vi "SetVIActivationEvent.vi"(8 "error in (no error)":errorcluster, 10 "VIActivation":refnum<user-event>, 11 "VI Activation in":refnum<class "VIActivation.lvclass">) -> (0 "error out":errorcluster, 3 "VI Activation out":refnum<class "VIActivation.lvclass">)   [LabVIEW 2021, in "VIActivation.lvlib" / "VIActivation.lvclass"]
uses:
  VIActivation.lvclass
  VIActivation.lvclass/VIActivation.ctl
  VIActivationEvents.ctl
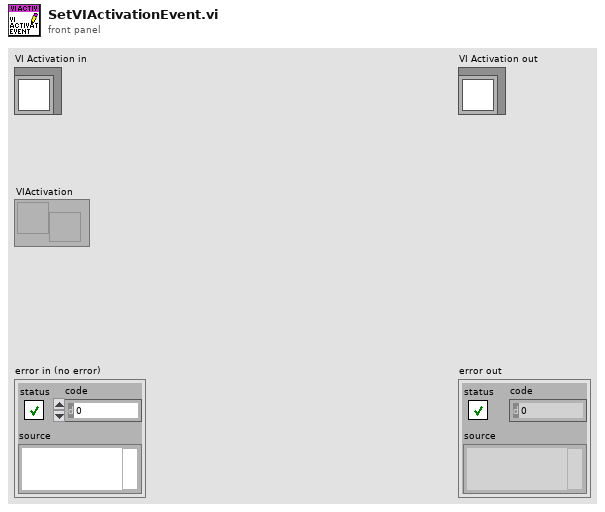
[diagram p1: front panel]
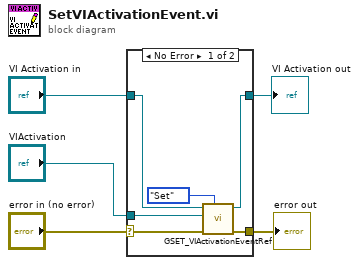
[diagram p0: block diagram]
diagram:
  n1 = case shown="No Error" "error in (no error)" {
    selector: "error in (no error)" -> [w11 w13]
    tunnel: [w10 w13] -> w4
    tunnel: [w9 w12] -> w2
    tunnel: "VI Activation in" -> [w8 w12]
    tunnel: "VIActivation" -> [w7 _]
    frame No Error {
      n2 = call "GSET_VIActivationEventRef.vi"("Action"=enum16{"Get", "Set"}."Set", "error in (no error)"=w11, "VIActivationEvent in"=w7, "Menu in"=w8) -> ("error out"=w10:errorcluster, "Menu out"=w9:refnum<class "VIActivation.lvclass">)  [unwired: 5 in, 1 out]
    }
    frame Error {
    }
  }
  "error out" <- w4
  "VI Activation out" <- w2
